vi "DUT_Wi_Fi_Name.vi"(8 "error in (no error)":errorcluster, 11 "String Input":string) -> (0 "error out":errorcluster, 3 "Wi_Fi Name":string)   [LabVIEW 2018]
uses:
  <vilib>/regexp/Match Regular Expression.xnode
panel:
  out "result string":string
  out "after match":string
  out "whole match":string
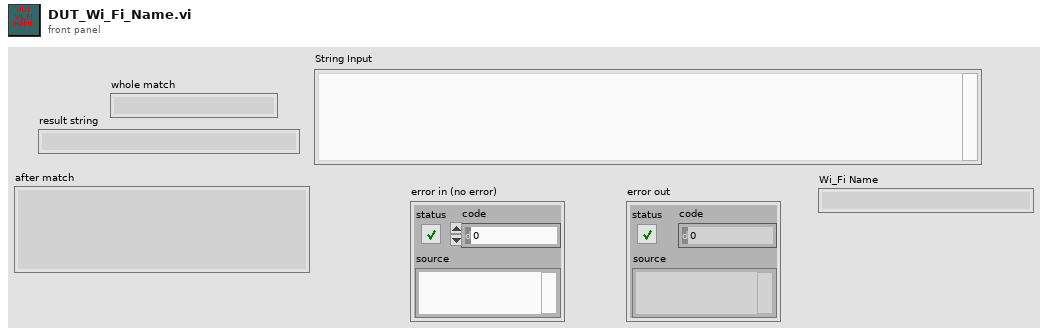
[diagram p1: front panel]
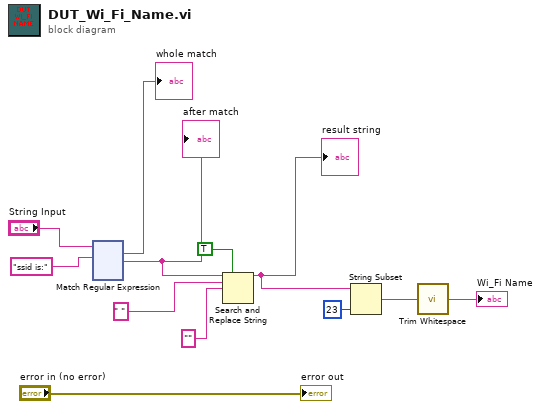
[diagram p0: block diagram]
diagram:
  n1 = xnode "Match Regular Expression"("input string"="String Input", "regular expression"="ssid is:") -> ("whole match"=→"whole match":string, "after match"=w9:string)  [unwired: 4 in, 3 out]
  "after match" <- w9
  n2 = Search and Replace String(replace all?=TRUE ("replace all? (F)"), input string=w9, search string=" ", replace string="" ("replace string (\"\")")) -> (result string=w6:string)  [unwired: 4 in, 3 out]
  "result string" <- w6
  n3 = String Subset(string=w6, length (rest)=23 ("length (rest)")) -> (substring=w2:string)  [unwired: 1 in]
  n4 = call <vilib>:"Trim Whitespace.vi"("string"=w2) -> ("trimmed string"=→"Wi_Fi Name":string)  [unwired: 1 in]
  "error out" <- "error in (no error)"
